vi "Update Status in Tree.vi"(6 "Worker Status":string, 8 "error in (no error)":errorcluster, 9 "DC_UID":T1, 10 "WID":string, 11 "Tree Ref":refnum<vi>) -> (0 "error out":errorcluster)   [LabVIEW 2017, in "Application Manager.lvclass"]
uses:
  Application Manager.lvclass
  Common VIs/DC_UID.ctl
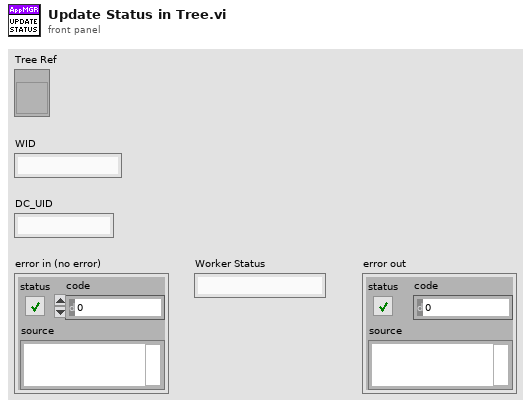
[diagram p1: front panel]
types:
  T1 = typedef "DC_UID.ctl" = string
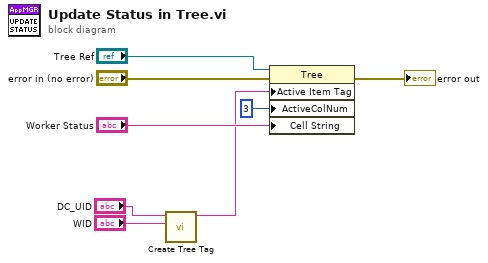
[diagram p0: block diagram]
diagram:
  n1 = call "Create Tree Tag.vi"("WID"="WID", "DC_UID"="DC_UID") -> ("Tree Tag"=w1:string)  [unwired: 9 in]
  n2 = property class="Tree"(reference="Tree Ref", error in="error in (no error)", "Active Item Tag"=w1, "ActiveColNum"=3 ("Active Cell:Active Column Number"), "Cell String"="Worker Status") -> (error out=→"error out":errorcluster)  [unwired: 1 out]
